vi "Amium PNS Grenzwerte pruefen.vi"(9 "Wert":dbl, 11 "Parameternamen PNS":T1=enum."Heizkreis 3") -> (0 "AbschMax":bool, 1 "AbschMin":bool, 2 "WarnMax":bool, 3 "WarnMin":bool, 5 "F.Br.":bool)   [LabVIEW 2020, in "Amium PNS.lvlib"]
uses:
  Amium PNS.lvlib
  PNS/Parameternamen PNS.ctl
  Aktion FGV Amium Daten.ctl
  PNS/PNS.lvlib
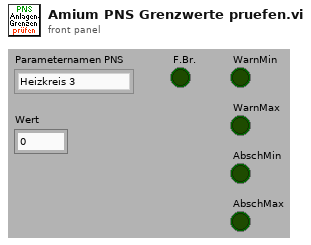
[diagram p1: front panel]
types:
  T1 = typedef "PNS.lvlib/Parameternamen PNS.ctl" = enum16{"Heizkreis 1", "Heizkreis 2", "Heizkreis 3", "Heizkreis 4", "Heizkreis 5", "Heizkreis 6", "Heizkreis 7", "Heizkreis 8"}
  T2 = typedef "Amium PNS.lvlib/Aktion FGV Amium Daten.ctl" = enum16{"lesen", "Komm Daten", "Daten", "Error", "Regler", "Grenzwerte", "laden", "speichern"}
  T3 = typedef "Amium PNS.lvlib/Amium Anlagengrenzwerte PNS.ctl" = cluster{"Filter:":T4, "Ventilplatte:":T4, "Heizleitung 1:":T4, "Heizleitung 2:":T4, "Heizleitung 3:":T4, "Heizleitung 4:":T4, "Heizleitung 5:":T4, "Heizleitung 6:":T4, "Heizleitung 7:":T4, "Heizleitung 8:":T4, "Heizleitung 9:":T4, "Heizleitung 10:":T4, "Heizleitung 11:":T4, "Heizleitung 12:":T4}
  T4 = typedef "Amium PNS.lvlib/Amium Anlagengrenzwerte-Parameter Anzeige.ctl" = cluster{"Sollwert":T5, "Warn-Min":T5, "Warn-Max":T5, "Abschalt-Min":T5, "Abschalt-Max":T5, "Regler":u16}
  T5 = typedef "Zahlen-Eingabefeld.ctl" = sgl
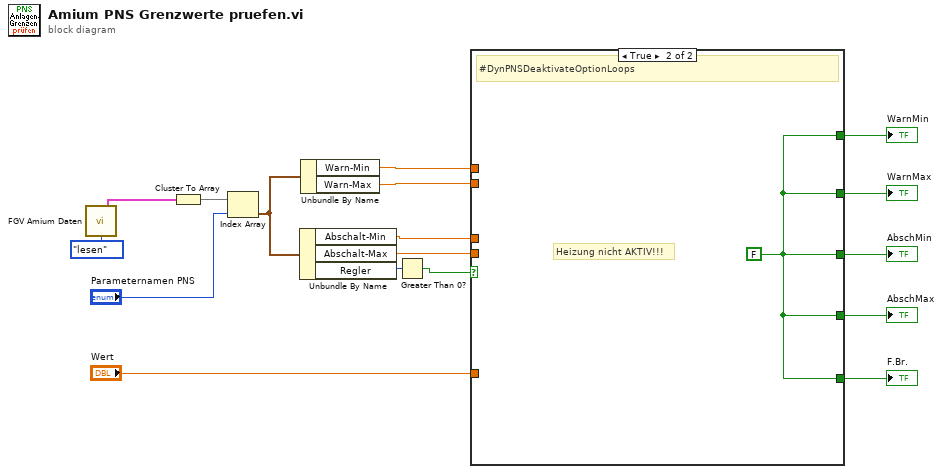
[diagram p0: block diagram]
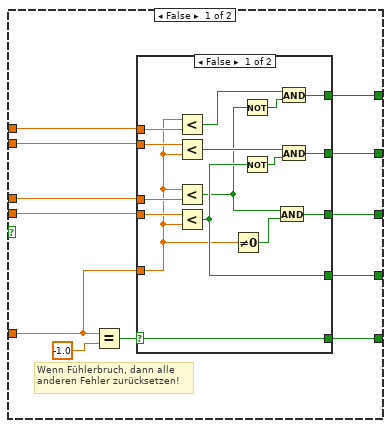
[diagram p2: hidden frame]
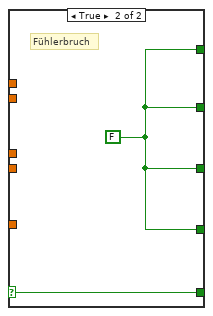
[diagram p3: hidden frame]
diagram:
  n1 = call "FGV Amium Daten.vi"("Aktion"=Aktion_FGV_Amium_Daten."lesen") -> ("Grenzwerte PNS"=w1:T3)  [unwired: 9 in, 5 out]
  n2 = Cluster To Array(cluster=w1) -> (array=w17:T4[])
  n3 = Index Array(array=w17, index="Parameternamen PNS") -> (element=w16:T4)
  n4 = Unbundle By Name(w16) -> ("Abschalt-Min"=w13:T5, "Abschalt-Max"=w12:T5, "Regler"=w4:u16)
  n5 = Unbundle By Name(w16) -> ("Warn-Min"=w15:T5, "Warn-Max"=w14:T5)
  n6 = Greater Than 0?(x=w4) -> (x > 0?=w3:bool)
  n7 = case shown="True" w3 {
    tunnel: w15 -> [w29 _]
    tunnel: w14 -> [w28 _]
    tunnel: w13 -> [w27 _]
    tunnel: w12 -> [w26 _]
    tunnel: [w25 w48] -> w11
    tunnel: [w24 w48] -> w10
    tunnel: [w23 w48] -> w9
    tunnel: [w22 w48] -> w8
    tunnel: [w21 w48] -> w7
    tunnel: "Wert" -> [w20 _]
    frame False {
      # "Wenn Fühlerbruch, dann alle \nanderen Fehler zurücksetzen!"
      n8 = Equal?(x=w20, y=-1.0) -> (x = y?=w19:bool)
      n9 = case shown="False" w19 {
        selector: w19 -> [w34 w47]
        tunnel: w29 -> [w45 _]
        tunnel: w28 -> [w44 _]
        tunnel: w27 -> [w43 _]
        tunnel: w26 -> [w42 _]
        tunnel: [w37 w46] -> w21
        tunnel: [w36 w46] -> w22
        tunnel: [w30 w46] -> w23
        tunnel: [w35 w46] -> w24
        tunnel: w20 -> [w33 _]
        tunnel: [w34 w47] -> w25
        frame False {
          n10 = Less?(x=w33, y=w45) -> (x < y?=w41:bool)
          n11 = Less?(x=w44, y=w33) -> (x < y?=w38:bool)
          n12 = Less?(x=w33, y=w43) -> (x < y?=w31:bool)
          n13 = Less?(x=w42, y=w33) -> (x < y?=w35:bool)
          n14 = Not Equal To 0?(x=w33) -> (x != 0?=w32:bool)
          n15 = Not(x=w31) -> (.not. x?=w40:bool)
          n16 = Not(x=w35) -> (.not. x?=w39:bool)
          n17 = And(x=w31, y=w32) -> (x .and. y?=w30:bool)
          n18 = And(x=w41, y=w40) -> (x .and. y?=w37:bool)
          n19 = And(x=w38, y=w39) -> (x .and. y?=w36:bool)
        }
        frame True {
          w46 = FALSE
          # "Fühlerbruch"
        }
      }
    }
    frame True {
      w48 = FALSE
      # "Heizung nicht AKTIV!!!"
      # "#DynPNSDeaktivateOptionLoops"
    }
  }
  "WarnMin" <- w7
  "WarnMax" <- w8
  "AbschMin" <- w9
  "AbschMax" <- w10
  "F.Br." <- w11
